vi "Set and Couple Channels.vi"(8 "error in (no error)":errorcluster, 9 "channels coupled (F : uncoupled)":bool, 10 "active channel (T : CH1)":bool=TRUE, 11 "VISA resource name":refnum<visa-resource-name>) -> (0 "error out":errorcluster, 3 "VISA resource name out":refnum<visa-resource-name>)   [LabVIEW 2018, in "Agilent 87XX Series.lvlib"]
doc: "This VI for the HP8753B Network Analyzer is used to set the active channel and used to couple and uncouple channels."
uses:
  Agilent 87XX Series.lvlib
panel:
  # "channel 1\nchannel 2"
  # "coupled\nuncoupled"
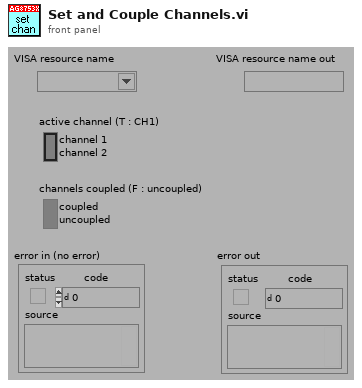
[diagram p1: front panel]
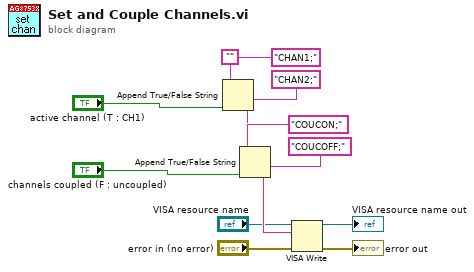
[diagram p0: block diagram]
diagram:
  n1 = Append True/False String(1:"active channel (T : CH1)", 2:"CHAN2;", 3:"CHAN1;", 4:"") -> (0:w7:string)
  n2 = Append True/False String(1:"channels coupled (F : uncoupled)", 2:"COUCOFF;", 3:"COUCON;", 4:w7) -> (0:w5:string)
  n3 = VISA Write(VISA resource name="VISA resource name", write buffer=w5, error in (no error)="error in (no error)") -> (VISA resource name out=→"VISA resource name out":refnum<visa-resource-name>, error out=→"error out":errorcluster)  [unwired: 1 out]
